vi "Set Task Outputs To String.vi"(0 "Sender":string, 1 "Task Outputs in":refnum<class "Task Outputs.lvclass">, 5 "Item Name":string, 7 "Generated Files":path[](array[path]), 9 "Build Specification Version":T1, 11 "Status":string="Built") -> (4 "data string":string)   [LabVIEW 2017, in "Message Interface.lvlib" / "Task Outputs.lvclass"]
uses:
  Task Outputs.lvclass
  C:/Users/Public/Documents/wc/BuildFarm/src/LabVIEW/vi.lib/BenjaminR/Build Farm/Classes/Message Interface/iMessage/iMessage.lvclass
  C:/Users/Public/Documents/wc/BuildFarm/src/LabVIEW/vi.lib/BenjaminR/Build Farm/Classes/Message Interface/Status/Status.lvclass
  <vilib>/AppBuilder/AB_API_Simple/Build Specification Version.ctl
  iMessage/iMessage.lvclass/iMessage.ctl
  Status/Status.lvclass/Status.ctl
  Task Outputs.lvclass/Task Outputs.ctl
  iMessage/Write Sender.vi
  Status/Write Item Name.vi
  Write Build Specification Version.vi
  Write Generated Files.vi
  iMessage/iMessage.lvclass
  <vilib>/AppBuilder/AB_API_Simple/NI_App_Builder_API.lvlib
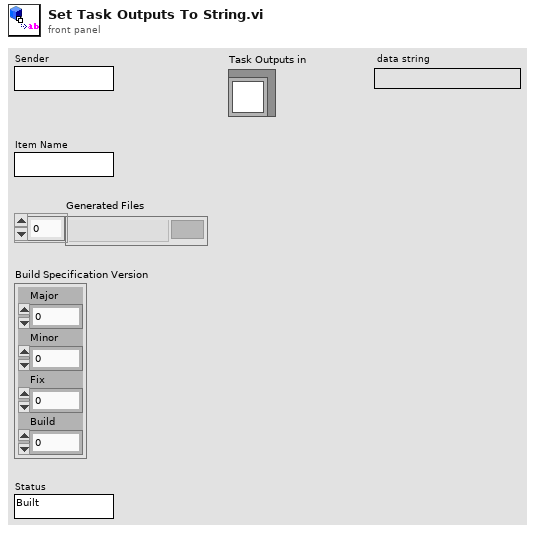
[diagram p1: front panel]
types:
  T1 = typedef "NI_App_Builder_API.lvlib/Build Specification Version.ctl" = cluster{"Major":u16, "Minor":u16, "Fix":u16, "Build":u16}
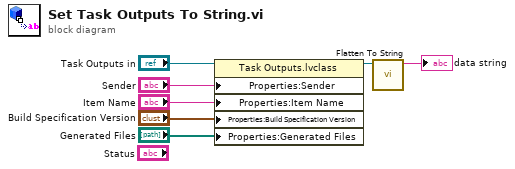
[diagram p0: block diagram]
diagram:
  n1 = property class="Task Outputs.lvclass"(reference="Task Outputs in", "Properties:Sender"="Sender", "Properties:Item Name"="Item Name", "Properties:Build Specification Version"="Build Specification Version", "Properties:Generated Files"="Generated Files") -> (reference out=w2:refnum<class "Task Outputs.lvclass">)  [unwired: 1 in, 1 out]
  n2 = call "Flatten To String.vi"("iMessage in"=w2) -> ("data string"=→"data string":string)  [unwired: 9 in, 1 out]
